vi "Untabify.vi"(0 "string in":string, 1 "spaces":i32=4) -> (2 "string out":string)   [LabVIEW 2014, in "Raspberry Pi Compatible Compiler for LabVIEW.lvlib" / "Python Functions.lvlib"]
uses:
  Python Functions.lvlib
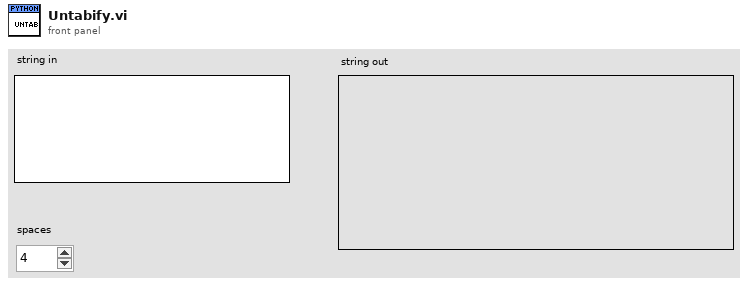
[diagram p1: front panel]
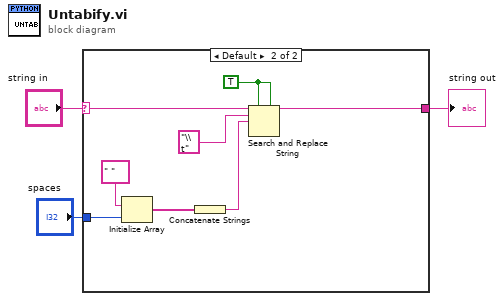
[diagram p0: block diagram]
diagram:
  n1 = case shown="Default" "string in" {
    selector: "string in" -> [_ w5]
    tunnel: [_ w4] -> w3
    tunnel: "spaces" -> [_ w8]
    frame "" {
    }
    frame Default {
      w11 = TRUE ("replace all? (F)")
      n2 = Initialize Array(" " ("String"), w8) -> (w6:string[])
      n3 = Concatenate Strings(w6) -> (w9:string)
      n4 = Search and Replace String(replace all?=w11, multiline?=w11, input string=w5, search string="\\t", replace string=w9) -> (result string=w4:string)  [unwired: 3 in, 3 out]
    }
  }
  "string out" <- w3
